vi "get Data Element.vi"(0 "LVx - Template Command in":refnum<class "REx - NART - Abort Receive.lvclass">, 11 "error in (no error)":errorcluster) -> (4 "LVx - Template Command out":refnum<class "REx - NART - Abort Receive.lvclass">, 6 "RX Response":T1, 15 "error out":errorcluster)   [LabVIEW 2011, in "ART2 Test Panel.lvlib" / "REx - NART - Abort Receive.lvclass"]
uses:
  REx - NART - Abort Receive.lvclass
  Components/ART2.llb/NART/Controls/Receive Response.ctl
  REx - NART - Abort Receive.lvclass/REx - NART - Abort Receive.ctl
  ART2 Test Panel.lvlib
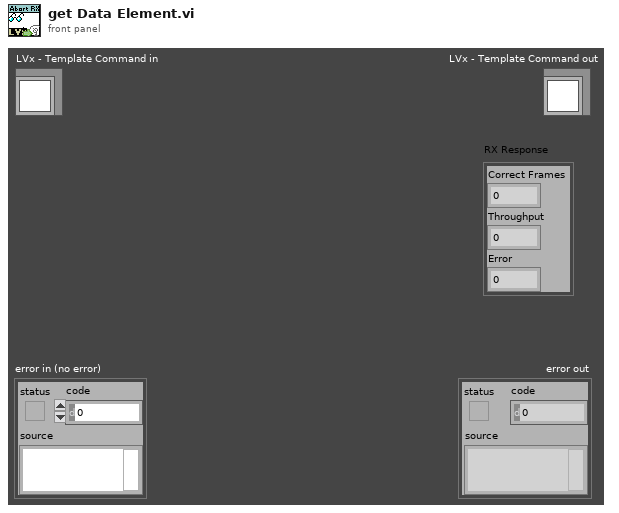
[diagram p1: front panel]
types:
  T1 = typedef "ART2 Test Panel.lvlib/Receive Response.ctl" = cluster{"Correct Frames":i32, "Throughput":i32, "Error":i32}
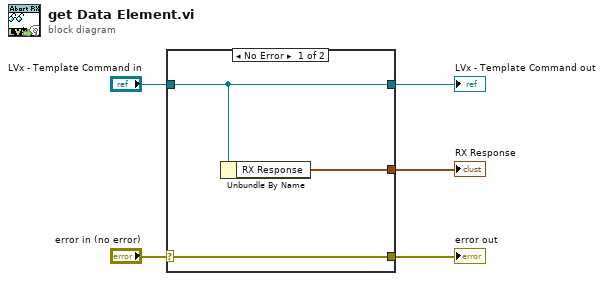
[diagram p0: block diagram]
diagram:
  n1 = case shown="No Error" "error in (no error)" {
    selector: "error in (no error)" -> [w8 w9]
    tunnel: [w8 w9] -> w4
    tunnel: [w6 w10] -> w2
    tunnel: "LVx - Template Command in" -> [w6 w10]
    tunnel: [w7 _] -> w1
    frame No Error {
      n2 = Unbundle By Name(w6) -> ("RX Response"=w7:T1)
    }
    frame Error {
    }
  }
  "error out" <- w4
  "LVx - Template Command out" <- w2
  "RX Response" <- w1
